vi "dfd_Get Coefficient of QMF Lattice.vi"(8 "error in (no error)":errorcluster, 9 "hm1":dbl[](array[numeric]), 10 "hm0":dbl[](array[numeric])) -> (0 "error out":errorcluster, 2 "am":dbl)   [LabVIEW 2017, in "NI_DigFilter_FilterBank.lvlib"]
doc: "computes lattice coefficients recursively."
uses:
  <vilib>/addons/Digital Filter Design/NI_DigFilter_FilterBank.lvlib
  <vilib>/Analysis/7linalg.llb/Solve Linear Equations (single right hand).vi
  <vilib>/Analysis/baseanly.llb/Solve Linear Equations By Cholesky.vi
  <vilib>/Analysis/baseanly.llb/Real Matrix to Compact Array.vi
  <vilib>/Analysis/baseanly.llb/Real Compact Tri-Matrix Linear Eqs.vi
  <vilib>/addons/Digital Filter Design/_Misc.llb/dfd_Error Handlers (Single).vi
  <vilib>/Analysis/7linalg.llb/Solve Linear Eqs (General).vi
  <vilib>/Analysis/7linalg.llb/Solve Linear Eqs (Gen, single right hand).vi
  <vilib>/addons/Digital Filter Design/NI_DigFilterLicensed.lvlib
  <vilib>/Analysis/NI_AALPro.lvlib
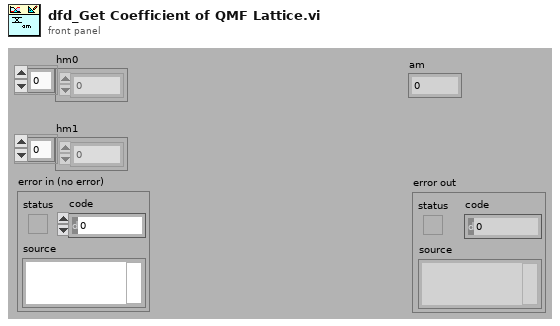
[diagram p1: front panel]
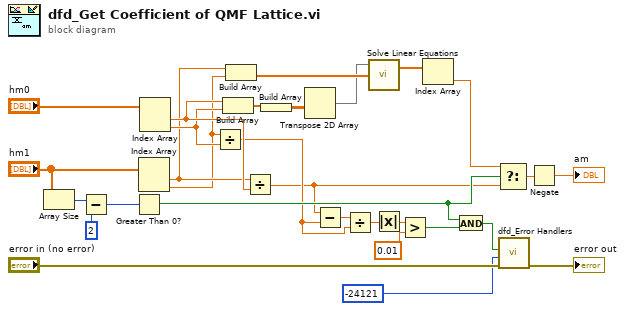
[diagram p0: block diagram]
diagram:
  n1 = Array Size(array="hm1") -> (size(s)=w20:i32)
  n2 = Subtract(x=w20, y=2) -> (x-y=w22:i32)
  n3 = Greater Than 0?(x=w22) -> (x > 0?=w23:bool)
  n4 = Index Array(array="hm1") -> (element #1=w14:dbl, element #2=w13:dbl)  [unwired: 2 in]
  n5 = Index Array(array="hm0") -> (element #1=w19:dbl, element #2=w18:dbl)  [unwired: 2 in]
  n6 = Divide(x=w13, y=w18) -> (x/y=w15:dbl)
  n7 = Build Array(w19, w18) -> (w12:dbl[])
  n8 = Build Array(w14, w13) -> (w11:dbl[])
  n9 = Divide(x=w14, y=w19) -> (x/y=w6:dbl)
  n10 = Build Array(w12) -> (w10:dbl[][])
  n11 = Transpose 2D Array(2D array=w10) -> (transposed array=w9:dbl[][])
  n12 = Subtract(x=w6, y=w15) -> (x-y=w5:dbl)
  n13 = Divide(x=w5, y=w15) -> (x/y=w3:dbl)
  n14 = call-poly <vilib>:"Solve Linear Equations.vi"("Known Vector"=w11, "Input Matrix"=w9) -> ("Solution Vector"=w8:dbl[])  [unwired: 1 in, 1 out]
  n15 = Absolute Value(x=w3) -> (abs(x)=w4:dbl)
  n16 = Greater?(x=w4, y=0.01) -> (0:w25:bool)
  n17 = Index Array(array=w8) -> (element=w7:dbl)  [unwired: 1 in]
  n18 = And(x=w23, y=w25) -> (x .and. y?=w2:bool)
  n19 = Select(t=w7, s=w23, f=w6) -> (s? t:f=w21:dbl)
  n20 = call-poly <vilib>:"dfd_Error Handlers.vi"("error in (no error)"="error in (no error)", "error code"=-24121 ("ERR_INVALID_FILTERBANK_OBJ"), "condition failed?"=w2) -> ("error out"=→"error out":errorcluster)  [unwired: 8 in]
  n21 = Negate(x=w21) -> (-x=→"am":dbl)
